vi "GetState_ServerIPPort.vi"(8 "error in (no error)":errorcluster caption="错误输入（无错误）", 11 "TCPServerClass输入":refnum<class "TCPServerClass.lvclass">) -> (0 "error out":errorcluster caption="错误输出", 2 "服务端识别":cluster{"本机IP":string, "本机端口":u16}, 3 "TCPServerClass输出":refnum<class "TCPServerClass.lvclass">)   [LabVIEW 2019, in "TCPServerClass.lvclass"]
uses:
  TCPServerClass.lvclass
  TCPServerClass.lvclass/TCPServerClass.ctl
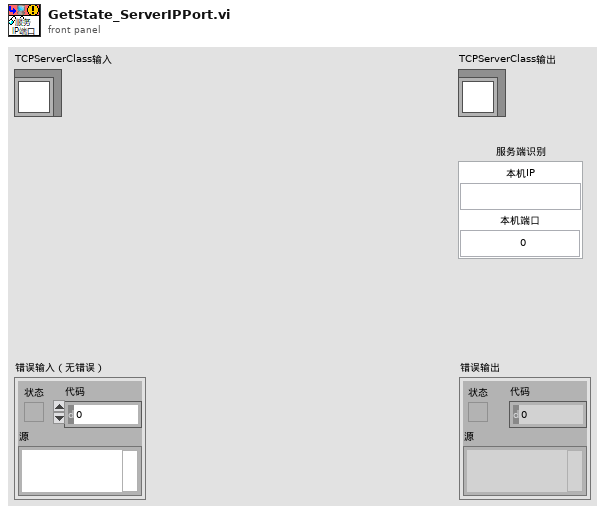
[diagram p1: front panel]
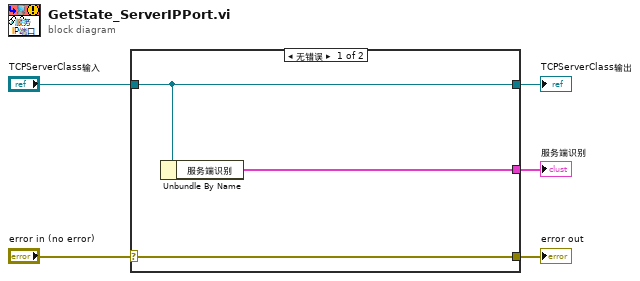
[diagram p0: block diagram]
diagram:
  n1 = case shown="无错误" "error in (no error)" {
    selector: "error in (no error)" -> [w8 w9]
    tunnel: [w8 w9] -> w4
    tunnel: [w7 w10] -> w2
    tunnel: "TCPServerClass输入" -> [w7 w10]
    tunnel: [w6 _] -> w1
    frame No Error {
      n2 = Unbundle By Name(w7) -> ("服务端识别"=w6:cluster{"本机IP":string, "本机端口":u16})
    }
    frame Error {
    }
  }
  "error out" <- w4
  "TCPServerClass输出" <- w2
  "服务端识别" <- w1
